vi "SCLN_OffComm.vi"(4 "Server Name":string) -> ()   [LabVIEW 2015]
uses:
  SCLN_RW_Select.ctl
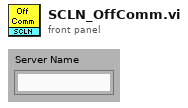
[diagram p1: front panel]
types:
  T1 = typedef "SCLN_RW_Select.ctl" = enum16{"Read", "Write"}
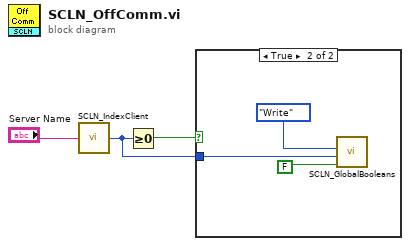
[diagram p0: block diagram]
diagram:
  n1 = call "SCLN_IndexClient.vi"("Server Name"="Server Name") -> ("Index"=w2:i32)
  n2 = Greater Or Equal To 0?(x=w2) -> (x >= 0?=w3:bool)
  n3 = case shown="True" w3 {
    tunnel: w2 -> [_ w4]
    frame False {
    }
    frame True {
      n4 = call "SCLN_GlobalBooleans.vi"("Write Value"=FALSE, "Element"=w4, "Operation"=SCLN_RW_Select."Write" ("GBL_RW")) -> ()  [unwired: 1 in, 2 out]
    }
  }
